vi "JKISM++ Get New State Notifier Event.vi"(8 "Error in":errorcluster caption="Error in (no error)", 11 "Name(\"\" to use uuid) in":string) -> (0 "Error out":errorcluster, 3 "New State Notifier Event":refnum<user-event>)   [LabVIEW 2014, in "JKI-State-Machine-Plus.lvlib"]
uses:
  JKI-State-Machine-Plus.lvlib
  _Support/_JKISMQFGVOPER.ctl
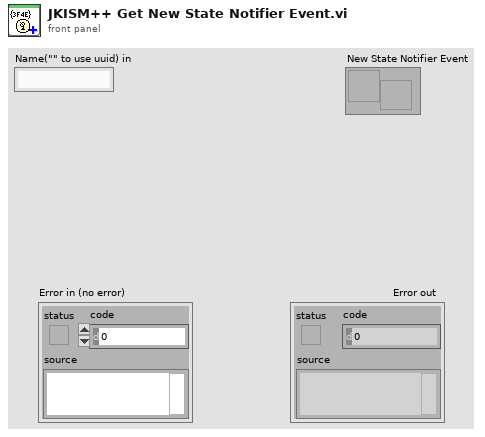
[diagram p1: front panel]
types:
  T1 = typedef "JKI-State-Machine-Plus.lvlib/_JKISMQFGVOPER.ctl" = enum16{"Get By Name", "List", "Check If Name Exists"}
  T2 = typedef "JKI-State-Machine-Plus.lvlib/_JKISMQ.ctl" = cluster{"Queue":refnum<queue>, "Locked Status":refnum<data-value>, "Stand Alone Mode":bool, "UserEvent":refnum<user-event>}
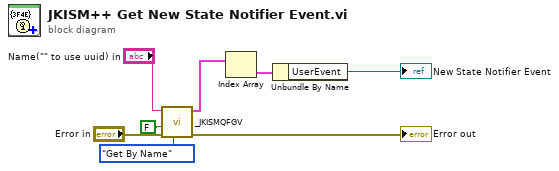
[diagram p0: block diagram]
diagram:
  n1 = call "_JKISMQFGV.vi"(6:_JKISMQFGVOPER."Get By Name", "Error in"="Error in", "create if not found? (T)"=FALSE, "Name(\"\" to use uuid) in"="Name(\"\" to use uuid) in") -> ("Error out"=→"Error out":errorcluster, "Array"=w3:T2[])  [unwired: 4 in, 2 out]
  n2 = Index Array(array=w3) -> (element=w2:T2)  [unwired: 1 in]
  n3 = Unbundle By Name(w2) -> ("UserEvent"=→"New State Notifier Event":refnum<user-event>)
